vi "Action Handler.vi"(8 "error in (no error)":errorcluster, 10 "Actions":T1, 11 "Core in":refnum<class "Core.lvclass">) -> (0 "error out":errorcluster, 3 "Core out":refnum<class "Core.lvclass">)   [LabVIEW 2019, in "Core.lvlib" / "Core.lvclass"]
uses:
  Core.lvclass
  Classes/States/MainStates/MainStates.lvclass
  Classes/States/MainStates/TypeDef/MainState.ctl
  ModuleAbstract/TypeDef/Module Actions.ctl
  ModuleAbstract/ModuleAbstract.lvclass
  <vilib>/ActorFramework/Message Enqueuer/Message Enqueuer.lvclass
  Classes/EventsAbstract/TypeDef/Event Actions.ctl
  Classes/EventsAbstract/EventsAbstract.lvclass
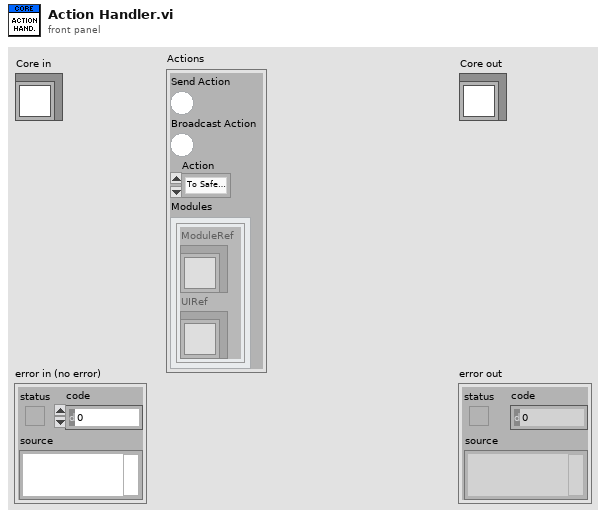
[diagram p1: front panel]
types:
  T1 = typedef "EventsAbstract.lvclass/Event Actions.ctl" = cluster{"Send Action":bool, "Broadcast Action":bool, "Action":T2, "Modules":cluster{"ModuleRef":refnum<class "Message Enqueuer.lvclass">, "UIRef":refnum<class "Message Enqueuer.lvclass">}[]}
  T2 = typedef "ModuleAbstract.lvlib/ModuleAbstract.lvclass/Module Actions.ctl" = enum16{"To Safe State", "Reset Safe State", "Close Module", "Close App"}
  T3 = typedef "MainState.ctl" = enum16{"Init", "Idle", "Safe Stop", "Normal Working", "Critical Error", "Closing"}
  T4 = cluster{"ModuleRef":refnum<class "Message Enqueuer.lvclass">, "UIRef":refnum<class "Message Enqueuer.lvclass">}[]
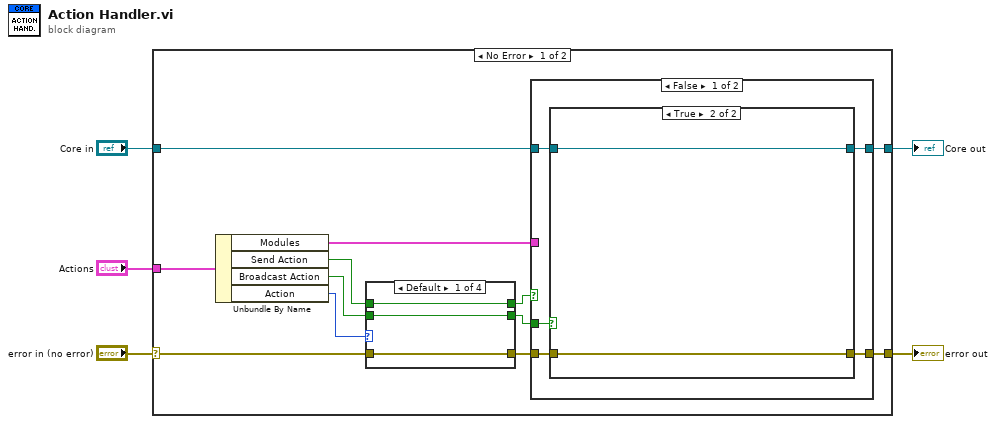
[diagram p0: block diagram]
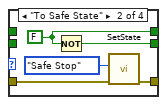
[diagram p4: hidden frame]
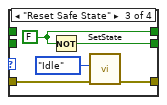
[diagram p5: hidden frame]
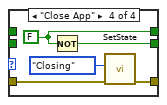
[diagram p6: hidden frame]
diagram:
  n1 = case shown="No Error" "error in (no error)" {
    selector: "error in (no error)" -> [w12 w48]
    tunnel: [w16 w48] -> w4
    tunnel: [w15 w47] -> w2
    tunnel: "Core in" -> [w14 w47]
    tunnel: "Actions" -> [w17 _]
    frame No Error {
      n2 = Unbundle By Name(w17) -> ("Modules"=w13:T4, "Send Action"=w8:bool, "Broadcast Action"=w9:bool, "Action"=w10:T2)
      n3 = case shown="Default" w10 {
        tunnel: w12 -> [w31 w36 w41 w46]
        tunnel: [w31 w34 w40 w45] -> w11
        tunnel: w9 -> [w30 _ _ _]
        tunnel: [w30 w32 w38 w42] -> w6
        tunnel: w8 -> [w29 _ _ _]
        tunnel: [w29 w33 w37 w43] -> w7
        frame Default {
        }
        frame "To Safe State" {
          w33 = FALSE
          n4 = Not(x=w33) -> (.not. x?=w32:bool)
          n5 = call "SetState.vi"("error in (no error)"=w36, "State"=MainState."Safe Stop") -> ("error out"=w34:errorcluster)  [unwired: 9 in]
        }
        frame "Reset Safe State" {
          w37 = FALSE
          n6 = Not(x=w37) -> (.not. x?=w38:bool)
          n7 = call "SetState.vi"("error in (no error)"=w41, "State"=MainState."Idle") -> ("error out"=w40:errorcluster)  [unwired: 9 in]
        }
        frame "Close App" {
          w43 = FALSE
          n8 = Not(x=w43) -> (.not. x?=w42:bool)
          n9 = call "SetState.vi"("error in (no error)"=w46, "State"=MainState."Closing") -> ("error out"=w45:errorcluster)  [unwired: 9 in]
        }
      }
      n10 = case shown="False" w7 {
        tunnel: [w22 w27] -> w16
        tunnel: w11 -> [w21 w27]
        tunnel: [w20 w28] -> w15
        tunnel: w14 -> [w19 w28]
        tunnel: w6 -> [w18 _]
        tunnel: w13 -> [_ _]
        frame False {
          n11 = case shown="True" w18 {
            tunnel: [w24 w26] -> w22
            tunnel: w21 -> [w24 w26]
            tunnel: [w23 w25] -> w20
            tunnel: w19 -> [w23 w25]
            frame False {
            }
            frame True {
            }
          }
        }
        frame True {
        }
      }
    }
    frame Error {
    }
  }
  "error out" <- w4
  "Core out" <- w2
